vi "Escape_Unescape Tests.vi"() -> ()   [LabVIEW 2011]
uses:
  JSON Scalar/JSON Scalar.lvclass
  JSON Scalar/Set String.vi
  JSON Scalar/Get as Text.vi
  Get Polymorphic/JSON GetSet.lvlib
panel:
  out "LabVIEW Text":string
  out "Lossless unflatten+flatten":bool
  in  "JSON stream":string="\"u-notation:  \\u00EE\\u002B\\u00CC\""
  out "String (normal display) after to/from JSON":string
  out "JSON (normal display)":string
  out "Lossless flatten+unflatten":bool
  in  "String ('\\' codes display)":string="Test \"quote\",\nnewline\rcarriage return and\ttab,\bbackspace,\fformfeed.\u0001\u0002"
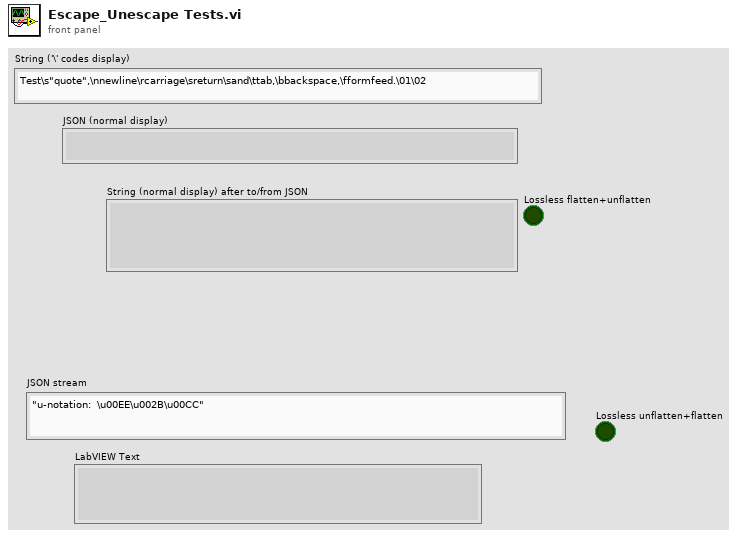
[diagram p1: front panel]
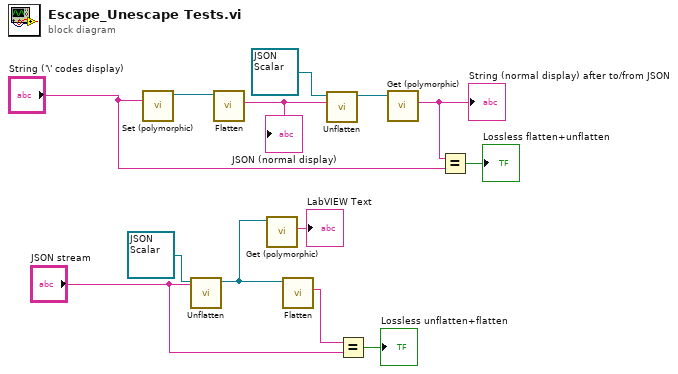
[diagram p0: block diagram]
diagram:
  n1 = call-poly "Set (polymorphic).vi"("String"="String ('\\' codes display)") -> ("JSON Scalar out"=w13:refnum<class "JSON Scalar.lvclass">)  [unwired: 9 in, 1 out]
  n2 = call-dynamic "Unflatten.vi"("JSON stream"="JSON stream", "JSON Scalar in"=refnum<class "JSON Scalar.lvclass"> refnum) -> ("JSON Scalar out"=w2:refnum<class "JSON Scalar.lvclass">)  [unwired: 6 in, 3 out]
  n3 = call-dynamic "Flatten.vi"("JSON Scalar in"=w13) -> ("String"=w10:string)  [unwired: 9 in, 1 out]
  "JSON (normal display)" <- w10
  n4 = call-poly "Get (polymorphic).vi"("JSON Scalar in"=w2) -> ("LabVIEW Text"=→"LabVIEW Text":string)  [unwired: 8 in, 2 out]
  n5 = call-dynamic "Flatten.vi"("JSON Scalar in"=w2) -> ("String"=w4:string)  [unwired: 9 in, 1 out]
  n6 = call-dynamic "Unflatten.vi"("JSON stream"=w10, "JSON Scalar in"=refnum<class "JSON Scalar.lvclass"> refnum) -> ("JSON Scalar out"=w12:refnum<class "JSON Scalar.lvclass">)  [unwired: 6 in, 3 out]
  n7 = Equal?(x=w4, y="JSON stream") -> (x = y?=→"Lossless unflatten+flatten":bool)
  n8 = call-poly "Get (polymorphic).vi"("JSON Scalar in"=w12) -> ("LabVIEW Text"=w9:string)  [unwired: 8 in, 2 out]
  "String (normal display) after to/from JSON" <- w9
  n9 = Equal?(x=w9, y="String ('\\' codes display)") -> (x = y?=→"Lossless flatten+unflatten":bool)
